vi "ZMQ Req Test.vi"() -> ()   [LabVIEW 2019, in "RemoteControl.ZMQ.lvlib" / "RemoteControl.ZMQ.lvclass"]
uses:
  RemoteControl.ZMQ.lvclass
  <vilib>/addons/zeromq/zmq_context.lvclass
  <vilib>/addons/zeromq/zmq_socket.lvclass
  <vilib>/addons/zeromq/socket_type.ctl
  <vilib>/addons/zeromq/zeromq.lvlib
  <vilib>/addons/zeromq/socket_options.ctl
  <userlib>/LevyLab/RemoteControl/RemoteControl/RemoteControl.lvclass
  C:/Program Files/National Instruments/LabVIEW 2019/user.lib/LevyLab/RemoteControl/RemoteControl/RemoteControl.lvclass
  C:/Program Files/National Instruments/LabVIEW 2019/vi.lib/JKI/JKI SMO/SMO/SMO.lvclass
panel:
  in  "milliseconds to wait":u32
  out "msg/s":dbl
  in  "stop":bool
  out "Data out":variant
  out "error out":errorcluster
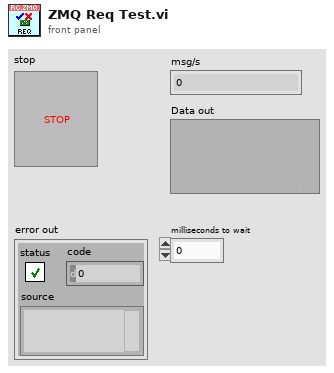
[diagram p1: front panel]
types:
  T1 = typedef "zeromq.lvlib/socket_options.ctl" = enum8{"NONE", "ZMQ_HWM", "<2>", "ZMQ_SWAP", "ZMQ_AFFINITY", "ZMQ_ROUTING_ID", "ZMQ_SUBSCRIBE", "ZMQ_UNSUBSCRIBE", "ZMQ_RATE", "ZMQ_RECOVERY_IVL", "ZMQ_MCAST_LOOP", "ZMQ_SNDBUF", "ZMQ_RCVBUF", "ZMQ_RCVMORE", "ZMQ_FD", "ZMQ_EVENTS", "ZMQ_TYPE", "ZMQ_LINGER", "ZMQ_RECONNECT_IVL", "ZMQ_BACKLOG", "ZMQ_RECOVERY_IVL_MSEC", "ZMQ_RECONNECT_IVL_MAX", "ZMQ_MAXMSGSIZE", "ZMQ_SNDHWM", "ZMQ_RCVHWM", "ZMQ_MULTICAST_HOPS", "<26>", "ZMQ_RCVTIMEO", "ZMQ_SNDTIMEO", "<29>", "<30>", "ZMQ_IPV4ONLY", "ZMQ_LAST_ENDPOINT", "ZMQ_ROUTER_MANDATORY", "ZMQ_TCP_KEEPALIVE", "ZMQ_TCP_KEEPALIVE_CNT", "ZMQ_TCP_KEEPALIVE_IDLE", "ZMQ_TCP_KEEPALIVE_INTVL", "ZMQ_TCP_ACCEPT_FILTER", "ZMQ_IMMEDIATE", "ZMQ_XPUB_VERBOSE", "ZMQ_ROUTER_RAW", "ZMQ_IPV6", "ZMQ_MECHANISM", "ZMQ_PLAIN_SERVER", "ZMQ_PLAIN_USERNAME", "ZMQ_PLAIN_PASSWORD", "ZMQ_CURVE_SERVER", "ZMQ_CURVE_PUBLICKEY", "ZMQ_CURVE_SECRETKEY", "ZMQ_CURVE_SERVERKEY", "ZMQ_PROBE_ROUTER", "ZMQ_REQ_CORRELATE", "ZMQ_REQ_RELAXED", "ZMQ_CONFLATE", "ZMQ_ZAP_DOMAIN", "ZMQ_ROUTER_HANDOVER", "ZMQ_TOS", "ZMQ_IPC_FILTER_PID", "ZMQ_IPC_FILTER_UID", "ZMQ_IPC_FILTER_GID", "ZMQ_CONNECT_ROUTING_ID", "ZMQ_GSSAPI_SERVER", "ZMQ_GSSAPI_PRINCIPAL", "ZMQ_GSSAPI_SERVICE_PRINCIPAL", "ZMQ_GSSAPI_PLAINTEXT", "ZMQ_HANDSHAKE_IVL", "<67>", "ZMQ_SOCKS_PROXY", "ZMQ_XPUB_NODROP", "ZMQ_BLOCKY", "ZMQ_XPUB_MANUAL", "ZMQ_XPUB_WELCOME_MSG", "ZMQ_STREAM_NOTIFY", "ZMQ_INVERT_MATCHING", "ZMQ_HEARTBEAT_IVL", "ZMQ_HEARTBEAT_TTL", "ZMQ_HEARTBEAT_TIMEOUT", "ZMQ_XPUB_VERBOSER", "ZMQ_CONNECT_TIMEOUT", "ZMQ_TCP_MAXRT", "ZMQ_THREAD_SAFE", "<82>", "<83>", "ZMQ_MULTICAST_MAXTPDU", "ZMQ_VMCI_BUFFER_SIZE", "ZMQ_VMCI_BUFFER_MIN_SIZE", "ZMQ_VMCI_BUFFER_MAX_SIZE", "ZMQ_VMCI_CONNECT_TIMEOUT", "ZMQ_USE_FD", "ZMQ_GSSAPI_PRINCIPAL_NAMETYPE", "ZMQ_GSSAPI_SERVICE_PRINCIPAL_NAMETYPE", "ZMQ_BINDTODEVICE", "ZMQ_ZAP_ENFORCE_DOMAIN", "ZMQ_LOOPBACK_FASTPATH", "ZMQ_METADATA", "ZMQ_MULTICAST_LOOP", "ZMQ_ROUTER_NOTIFY"}
  T2 = typedef "zeromq.lvlib/socket_type.ctl" = enum8{"ZMQ_PAIR", "ZMQ_PUB", "ZMQ_SUB", "ZMQ_REQ", "ZMQ_REP", "ZMQ_DEALER", "ZMQ_ROUTER", "ZMQ_PULL", "ZMQ_PUSH", "ZMQ_XPUB", "ZMQ_XSUB", "ZMQ_STREAM", "ZMQ_SERVER", "ZMQ_CLIENT", "ZMQ_RADIO", "ZMQ_DISH", "ZMQ_GATHER", "ZMQ_SCATTER", "ZMQ_DGRAM"}
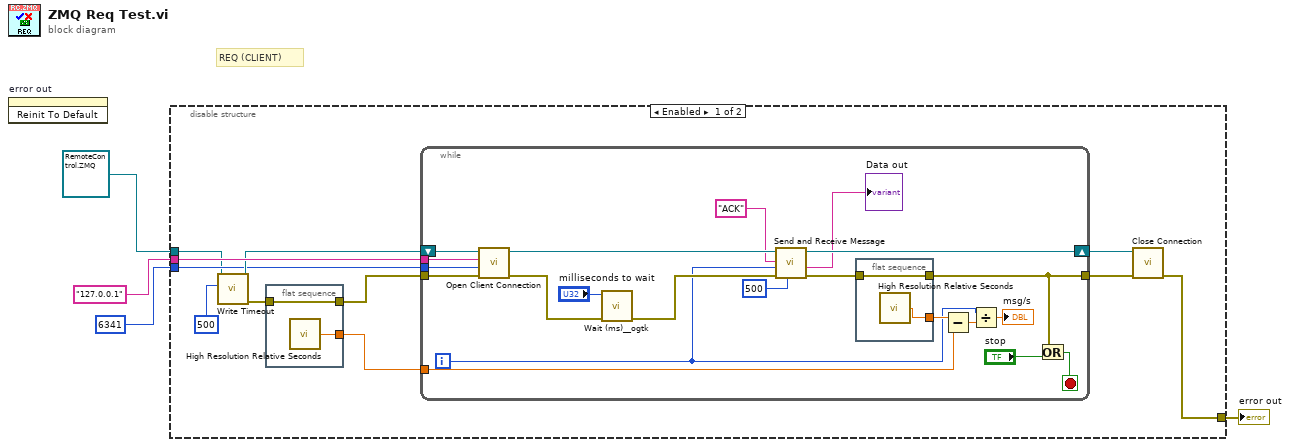
[diagram p0: block diagram]
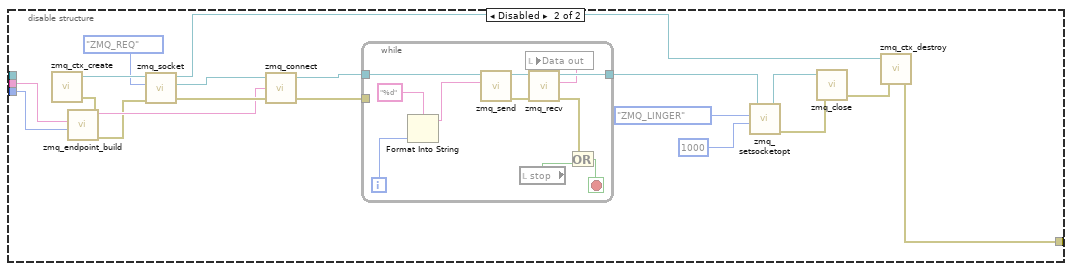
[diagram p2: hidden frame]
diagram:
  # "REQ (CLIENT)"
  n1 = invoke on="error out" class="Clust (strict)" method="Reinit To Default"() -> ()  [unwired: 3 in, 3 out]
  n2 = disable-structure shown="Enabled" {
    disable-tunnel: [w13 w42] -> w4
    disable-tunnel: "127.0.0.1" ("Address") -> [w11 w53]
    disable-tunnel: u16 6341 ("Port") -> [w9 w54]
    disable-tunnel: refnum<class "RemoteControl.ZMQ.lvclass"> refnum ("RemoteControl.ZMQ.lvlib:RemoteControl.ZMQ.lvclass") -> [w5 _]
    frame Enabled {
      n3 = call <userlib>:"Write Timeout.vi"("timeout (ms) [500]"=500 ("timeout in ms (100)"), "RemoteControl in"=w5) -> ("error out"=w8:errorcluster, "RemoteControl out"=w10:refnum<class "RemoteControl.ZMQ.lvclass">)  [unwired: 8 in]
      n4 = flat-sequence {
        tunnel: [w17] -> w6
        tunnel: w8 -> [w17]
        tunnel: [w16] -> w7
        frame #0 {
          n5 = call <vilib>:"High Resolution Relative Seconds.vi"() -> ("relative seconds"=w16:dbl)
        }
      }
      n6 = while {
        tunnel: [w29] -> w14
        tunnel: w6 -> [w27]
        tunnel: w7 -> [w32]
        shift-right: [w38] -> w15
        shift-left: w10 -> [w28]
        tunnel: w9 -> [w26]
        tunnel: w11 -> [w25]
        i -> [w21]
        stop <- w34 stop-if-true
        n7 = call-dynamic "Open Client Connection.vi"("error in (no error)"=w27, "port"=w26, "address"=w25, "RemoteControl.ZMQ in"=w28) -> ("error out"=w24:errorcluster, "RemoteControl.ZMQ out"=w22:refnum<class "RemoteControl.ZMQ.lvclass">)  [unwired: 6 in]
        n8 = call <userlib>:"Wait (ms)__ogtk.vi"("error in (no error)"=w24, "milliseconds to wait"="milliseconds to wait") -> ("error out"=w23:errorcluster)  [unwired: 8 in, 1 out]
        n9 = call-dynamic "Send and Receive Message.vi"("timeout (ms) [500]"=500, "error in (no error)"=w23, "Data"=w21, "Command"="ACK", "RemoteControl in"=w22) -> ("error out"=w35:errorcluster, "Data out"=→"Data out":string, "RemoteControl out"=w38:refnum<class "RemoteControl.ZMQ.lvclass">)  [unwired: 3 in, 1 out]
        n10 = flat-sequence {
          tunnel: [w40] -> w29
          tunnel: w35 -> [w40]
          tunnel: [w39] -> w33
          frame #0 {
            n11 = call <vilib>:"High Resolution Relative Seconds.vi"() -> ("relative seconds"=w39:dbl)
          }
        }
        n12 = Subtract(x=w33, y=w32) -> (x-y=w31:dbl)
        n13 = Divide(x=w21, y=w31) -> (x/y=→"msg/s":dbl)
        n14 = Or(x=w29, y="stop") -> (x .or. y?=w34:bool)
      }
      n15 = call-dynamic "Close Connection.vi"("error in (no error)"=w14, "RemoteControl.ZMQ in"=w15) -> ("error out"=w13:errorcluster)  [unwired: 8 in, 1 out]
    }
    frame Disabled {
      n16 = call <vilib>:"zmq_ctx_create.vi"() -> ("error out"=w50:errorcluster, "context out"=w57:refnum<class "zmq_context.lvclass">)  [unwired: 4 in]
      n17 = call <vilib>:"zmq_endpoint_build.vi"("error in"=w50, "port"=w54, "address"=w53) -> ("error out"=w49:errorcluster, "endpoint"=w55:string)  [unwired: 2 in, 1 out]
      n18 = call <vilib>:"zmq_socket.vi"("error in"=w49, "socket type"=socket_type."ZMQ_REQ", "context in"=w57) -> ("error out"=w59:errorcluster, "socket out"=w58:refnum<class "zmq_socket.lvclass">, "context out"=w43:refnum<class "zmq_context.lvclass">)  [unwired: 2 in]
      n19 = call <vilib>:"zmq_connect.vi"("error in"=w59, "endpoint"=w55, "socket in"=w58) -> ("error out"=w52:errorcluster, "socket out"=w51:refnum<class "zmq_socket.lvclass">)  [unwired: 1 in]
      n20 = while {
        tunnel: w52 -> [_]
        tunnel: w51 -> [w70]
        tunnel: [w63] -> w46
        i -> [w66]
        stop <- w64 stop-if-true
        n21 = Format Into String(format string="%d" ("Command"), w66) -> (resulting string=w60:string)  [unwired: 2 in, 1 out]
        n22 = call <vilib>:"zmq_send.vi"("data"=w60, "socket in"=w70) -> ("error out"=w69:errorcluster, "socket out"=w68:refnum<class "zmq_socket.lvclass">)  [unwired: 5 in]
        n23 = local read "stop"() -> (w65:bool)
        n24 = call <vilib>:"zmq_recv.vi"("error in"=w69, "socket in"=w68) -> ("error out"=w61:errorcluster, "data"=w62:string, "socket out"=w63:refnum<class "zmq_socket.lvclass">)  [unwired: 3 in, 2 out]
        n25 = local write "Data out"(w62) -> ()
        n26 = Or(x=w61, y=w65) -> (x .or. y?=w64:bool)
      }
      n27 = call <vilib>:"zmq_setsocketopt.vi"("value"=1000, "option"=socket_options."ZMQ_LINGER", "socket in"=w46) -> ("error out"=w45:errorcluster, "socket out"=w47:refnum<class "zmq_socket.lvclass">)  [unwired: 3 in]
      n28 = call <vilib>:"zmq_close.vi"("error in"=w45, "socket"=w47) -> ("error out"=w44:errorcluster)  [unwired: 3 in]
      n29 = call <vilib>:"zmq_ctx_destroy.vi"("error in"=w44, "context in"=w43) -> ("error out"=w42:errorcluster)  [unwired: 3 in]
    }
  }
  "error out" <- w4
